vi "Generate Signature.vi"(4 "consumer secret":string, 5 "Signature Method":T2=enum."HMAC-SHA1", 6 "token secret":string, 7 "HTTP Method":T3, 8 "error in (no error)":errorcluster, 10 "Parameters":T1[](array[typedef]), 11 "Base URL":string) -> (0 "error out":errorcluster, 2 "Signature":string)   [LabVIEW 2011, in "i3-oauth.lvlib"]
uses:
  i3-oauth.lvlib
  Controls/HTTP Method.ctl
  Controls/Signature Method.ctl
  Controls/key-value-pairs.ctl
  i3-oauth-dependencies/labviewencryption/hash-types.ctl
  i3-oauth-dependencies/i3-oauth-dependencies.lvlib
panel:
  out "Signature Base string":string
  out "Parameter string":string
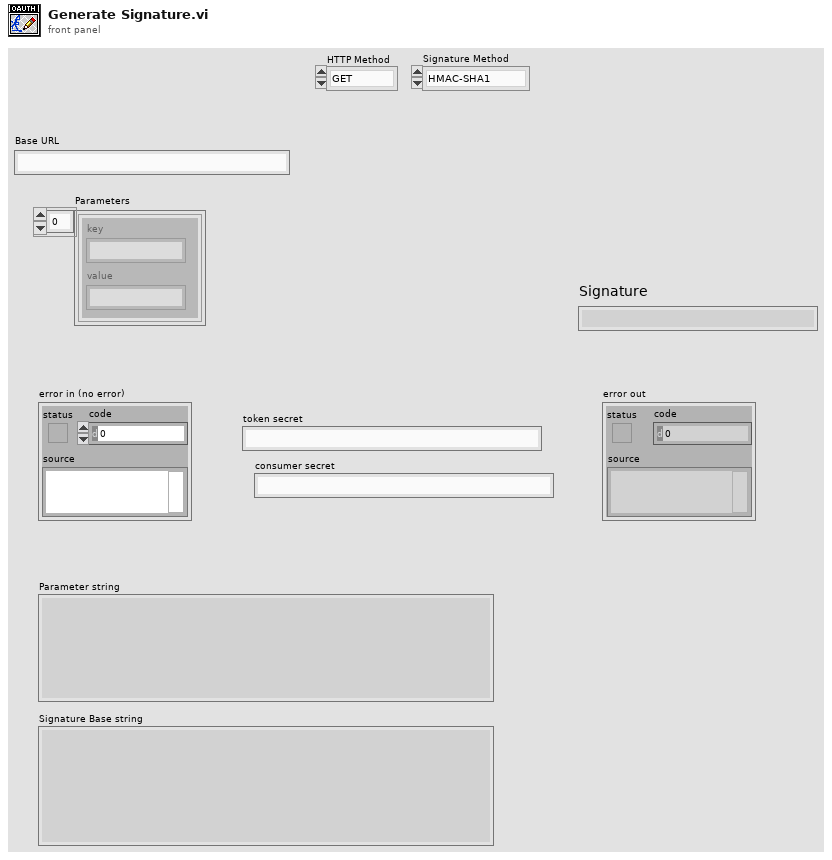
[diagram p1: front panel]
types:
  T1 = typedef "i3-oauth.lvlib/key-value-pairs.ctl" = cluster{"key":string, "value":string}
  T2 = typedef "i3-oauth.lvlib/Signature Method.ctl" = enum16{"HMAC-MD5", "HMAC-SHA1", "HMAC-SHA224", "HMAC-SHA256", "HMAC-SHA384", "HMAC-SHA512"}
  T3 = typedef "i3-oauth.lvlib/HTTP Method.ctl" = enum16{"GET", "POST", "PUT", "DELETE"}
  T4 = typedef "i3-oauth-dependencies.lvlib/hash-types.ctl" = enum16{"MD5", "SHA-1", "SHA-224", "SHA-256", "SHA-384", "SHA-512"}
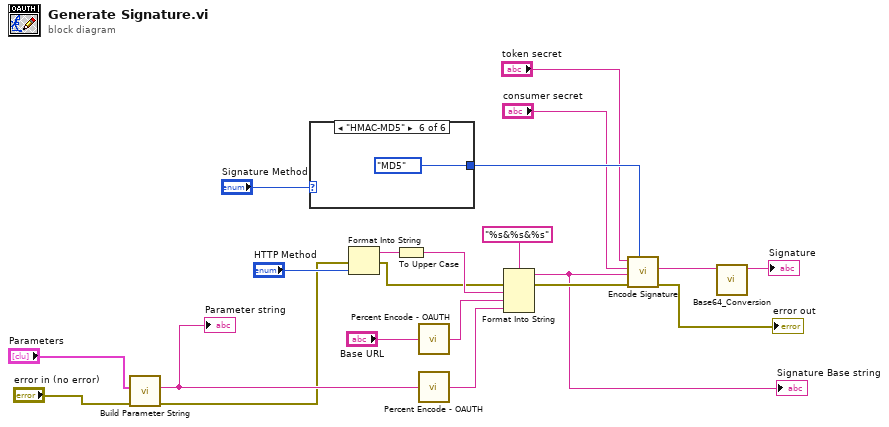
[diagram p0: block diagram]
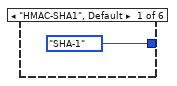
[diagram p2: hidden frame]
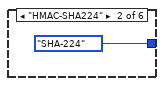
[diagram p3: hidden frame]
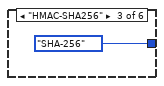
[diagram p4: hidden frame]
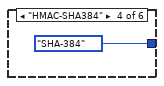
[diagram p5: hidden frame]
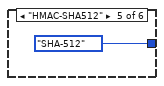
[diagram p6: hidden frame]
diagram:
  n1 = call "Build Parameter String.vi"("error in (no error)"="error in (no error)", "Parameters"="Parameters") -> ("error out"=w1:errorcluster, "Parameter String"=w15:string)  [unwired: 8 in]
  "Parameter string" <- w15
  n2 = case shown="\"HMAC-MD5\"" "Signature Method" {
    tunnel: [hash-types."SHA-1" ("HASH-method 2") hash-types."SHA-224" ("HASH-method 2") hash-types."SHA-256" ("HASH-method 2") hash-types."SHA-384" ("HASH-method 2") hash-types."SHA-512" ("HASH-method 2") hash-types."MD5" ("HASH-method 2")] -> w8
    frame "HMAC-SHA1", Default {
    }
    frame "HMAC-SHA224" {
    }
    frame "HMAC-SHA256" {
    }
    frame "HMAC-SHA384" {
    }
    frame "HMAC-SHA512" {
    }
    frame "HMAC-MD5" {
    }
  }
  n3 = Format Into String(error in=w1, "HTTP Method") -> (resulting string=w9:string, error out=w2:errorcluster)  [unwired: 2 in]
  n4 = To Upper Case(1:w9) -> (0:w20:string)
  n5 = call "Percent Encode - OAUTH.vi"("unescaped string in"="Base URL") -> ("escaped string out"=w18:string)
  n6 = call "Percent Encode - OAUTH.vi"("unescaped string in"=w15) -> ("escaped string out"=w17:string)
  n7 = Format Into String(format string="%s&%s&%s", error in=w2, w20, w18, w17) -> (resulting string=w5:string, error out=w13:errorcluster)  [unwired: 1 in]
  "Signature Base string" <- w5
  n8 = call "Encode Signature.vi"("HASH-method"=w8, "error in (no error)"=w13, "Signature Base string"=w5, "consumer secret"="consumer secret", "token secret"="token secret") -> ("error out"=→"error out":errorcluster, "Encoded Signature"=w12:string)  [unwired: 5 in]
  n9 = call "Base64_Conversion.vi"("String"=w12) -> ("Base64 String"=→"Signature":string)  [unwired: 10 in]
